vi "Move constant speed.vi"(10 "Enum":T1(ring), 11 "speed":i32) -> ()   [LabVIEW 2018]
panel:
  out "br":i32
  out "bl":i32
  out "fr":i16
  out "fl":i32
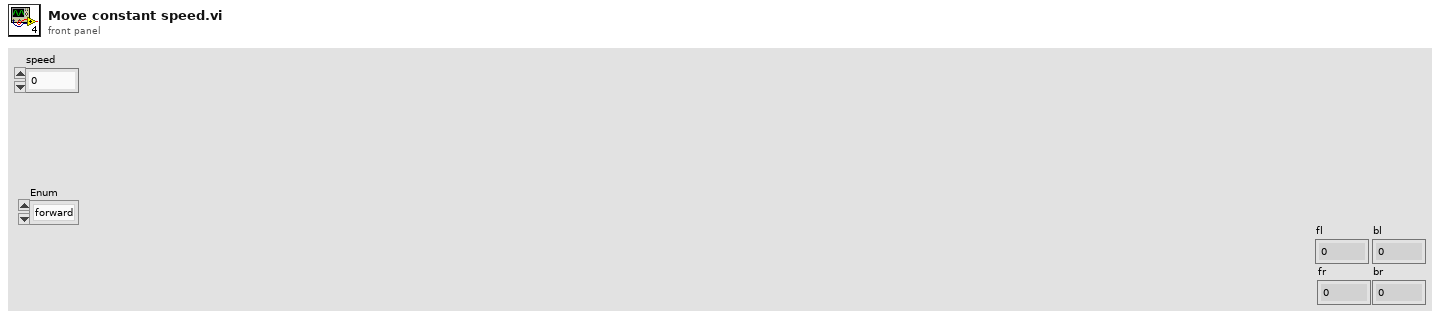
[diagram p1: front panel]
types:
  T1 = enum16{"forward", "backward", "left", "right", "rotate left", "rotate right"}
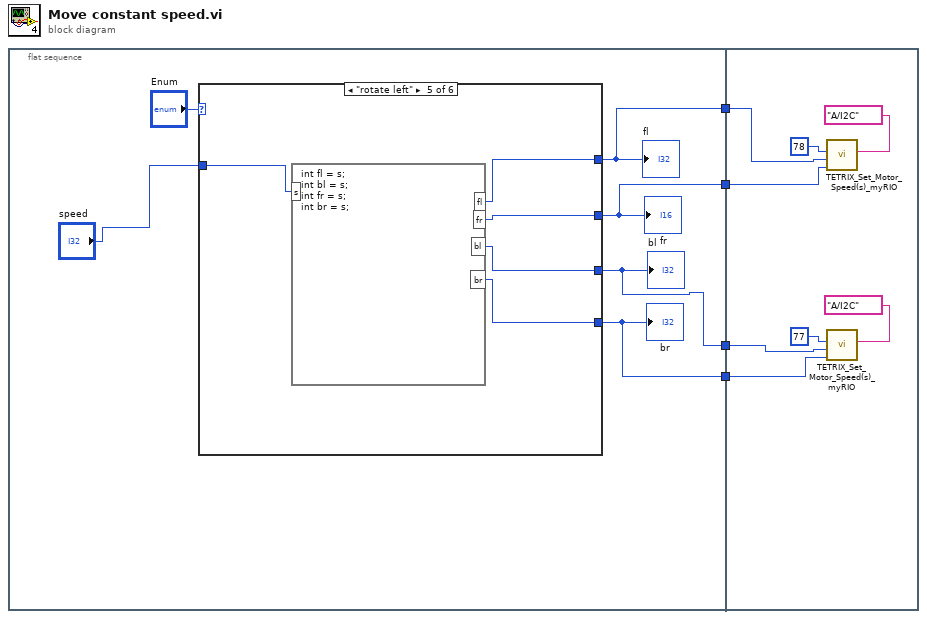
[diagram p0: block diagram]
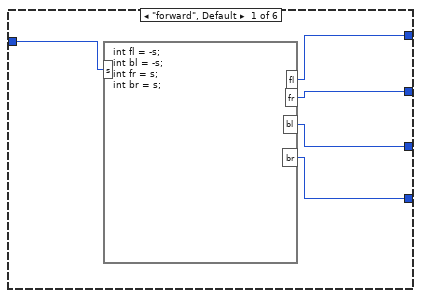
[diagram p2: hidden frame]
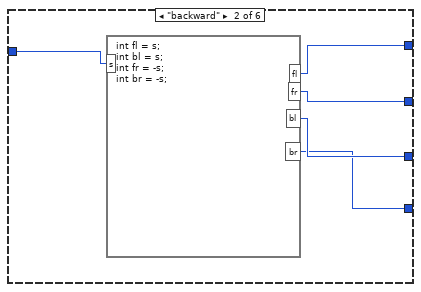
[diagram p3: hidden frame]
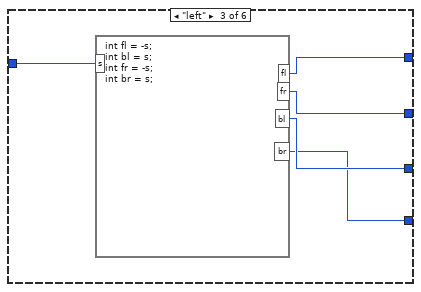
[diagram p4: hidden frame]
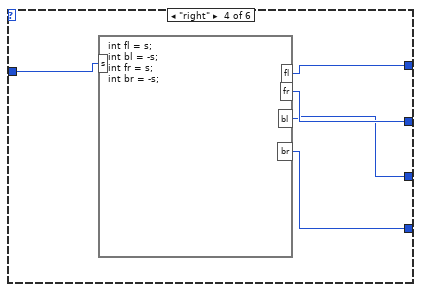
[diagram p5: hidden frame]
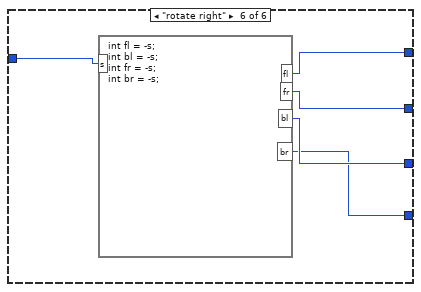
[diagram p6: hidden frame]
diagram:
  n1 = flat-sequence {
    tunnel: [w8] -> w4
    tunnel: [w7] -> w3
    tunnel: [w6] -> w2
    tunnel: [w5] -> w1
    tunnel: w4 -> [w44]
    tunnel: w3 -> [w43]
    tunnel: w2 -> [w42]
    tunnel: w1 -> [w41]
    frame #0 {
      n2 = case shown="\"rotate left\"" "Enum" {
        tunnel: "speed" -> [w15 w16 w25 w30 w35 w40]
        tunnel: [w14 w20 w24 w29 w34 w39] -> w8
        tunnel: [w13 w19 w23 w28 w33 w38] -> w7
        tunnel: [w12 w18 w22 w27 w32 w37] -> w6
        tunnel: [w11 w17 w21 w26 w31 w36] -> w5
        frame "forward", Default {
          n3 = formula code="int fl = -s;\nint bl = -s;\nint fr = s;\nint br = s;"("s"=w15) -> ("fl"=w14:i32, "fr"=w13:i32, "bl"=w12:i32, "br"=w11:i32)
        }
        frame "backward" {
          n4 = formula code="int fl = s;\nint bl = s;\nint fr = -s;\nint br = -s;"("s"=w16) -> ("fl"=w20:i32, "fr"=w19:i32, "bl"=w18:i32, "br"=w17:i32)
        }
        frame "left" {
          n5 = formula code="int fl = -s;\nint bl = s;\nint fr = -s;\nint br = s;"("s"=w25) -> ("fl"=w24:i32, "fr"=w23:i32, "bl"=w22:i32, "br"=w21:i32)
        }
        frame "right" {
          n6 = formula code="int fl = s;\nint bl = -s;\nint fr = s;\nint br = -s;"("s"=w30) -> ("fl"=w29:i32, "fr"=w28:i32, "bl"=w27:i32, "br"=w26:i32)
        }
        frame "rotate left" {
          n7 = formula code="int fl = s;\nint bl = s;\nint fr = s;\nint br = s;"("s"=w35) -> ("fl"=w34:i32, "fr"=w33:i32, "bl"=w32:i32, "br"=w31:i32)
        }
        frame "rotate right" {
          n8 = formula code="int fl = -s;\nint bl = -s;\nint fr = -s;\nint br = -s;"("s"=w40) -> ("fl"=w39:i32, "fr"=w38:i32, "bl"=w37:i32, "br"=w36:i32)
        }
      }
      "fl" <- w8
      "fr" <- w7
      "bl" <- w6
      "br" <- w5
    }
    frame #1 {
      n9 = call <vilib>:"TETRIX_Set_Motor_Speed(s)_myRIO.vi"("myRIO MXP Port A/B"=tag "A/I2C", "Motor 2 Speed (Degrees per second). Sign (+/-)  sets direction."=w43, "Motor 1 Speed (Degrees per second). Sign (+/-)  sets direction."=w44, "Controller ID#  (I2C Address)"=u8 78) -> ()  [unwired: 3 in, 1 out]
      n10 = call <vilib>:"TETRIX_Set_Motor_Speed(s)_myRIO.vi"("myRIO MXP Port A/B"=tag "A/I2C", "Motor 2 Speed (Degrees per second). Sign (+/-)  sets direction."=w41, "Motor 1 Speed (Degrees per second). Sign (+/-)  sets direction."=w42, "Controller ID#  (I2C Address)"=u8 77) -> ()  [unwired: 3 in, 1 out]
    }
  }
